vi "Temperature Limit.vi"(3 "Limite supérieure":dbl=80.0 format="%.2f", 4 "delta t (ms)":u32=400 min=50 max=2000 step=50, 5 "Points à acquérir":i32=75 min=20 max=500) -> ()   [LabVIEW 2013]
doc: "Ce VI simule l'acquisition de température, trace la température et notifie l'utilisateur si la température dépasse la limite."
panel:
  out "Limite dépassée":bool
  in  "Abandonner":bool
  out "Température":cluster{"Temperature":dbl, "High Limit":dbl}(graph)
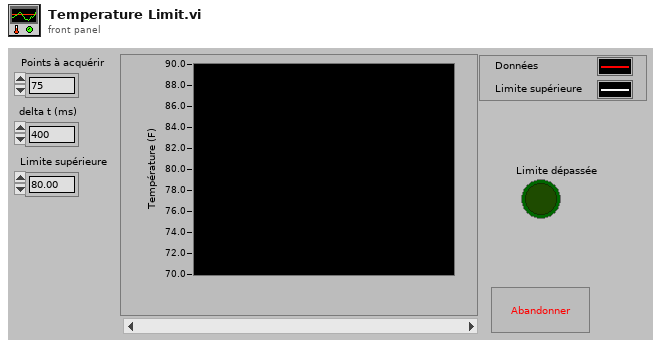
[diagram p1: front panel]
types:
  T1 = cluster{"Température":dbl, "Limite supérieure":dbl}
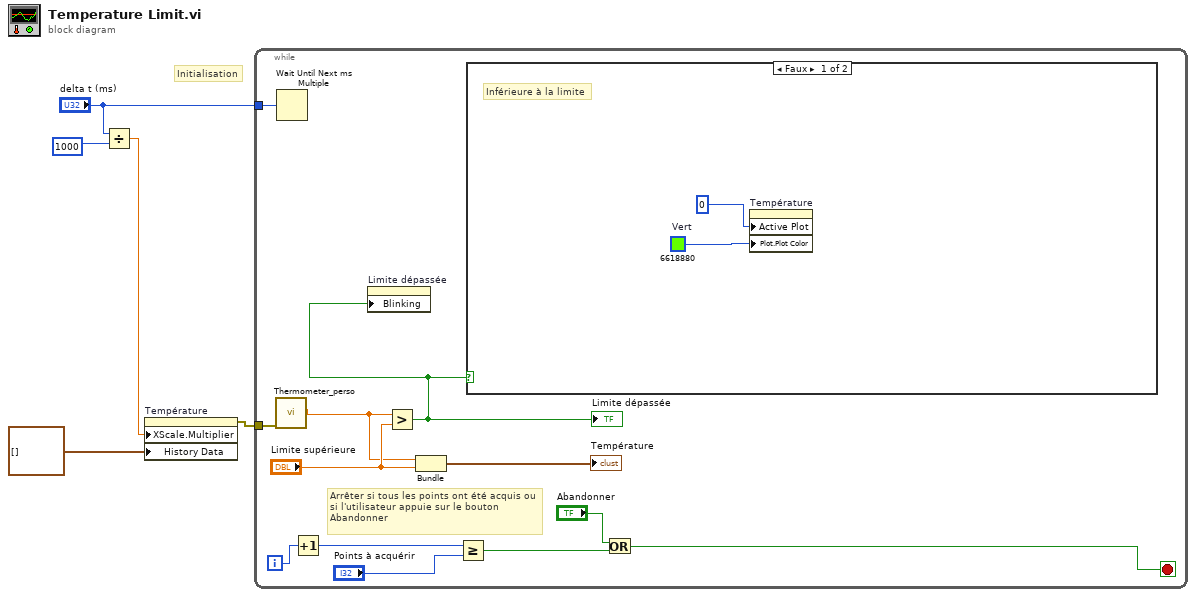
[diagram p0: block diagram]
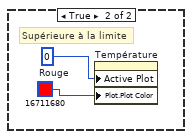
[diagram p2: hidden frame]
diagram:
  # "Initialisation"
  n1 = Divide(x="delta t (ms)", y=1000) -> (x/y=w3:dbl)
  n2 = property on="Température" class="GraphDér (strict)"("XScale.Multiplier"=w3, "History Data"=cluster{"Temperature":dbl, "High Limit":dbl}[] [] ("Données d'historique")) -> (error out=w2:errorcluster)  [unwired: 2 in, 1 out]
  n3 = while "Boucle While" {
    tunnel: "delta t (ms)" -> [w9]
    tunnel: w2 -> [w7]
    i -> [w16]
    stop <- w10 stop-if-true
    # "Supérieure à la limite"
    # "Arrêter si tous les points ont été acquis ou si l'utilisateur appuie sur le bouton Abandonner"
    n4 = call "Thermometer_perso.vi"("entrée d'erreur (pas d'erreur)"=w7) -> ("Température"=w8:dbl)  [unwired: 9 in, 1 out]
    n5 = Wait Until Next ms Multiple ("Structure Séquence empilée")(millisecond multiple=w9) -> ()  [unwired: 1 out]
    n6 = Increment ("Incrémenter")(x=w16) -> (x+1=w14:i32)
    n7 = Greater? ("Déplacer")(x=w8, y="Limite supérieure") -> (0:w6:bool)
    "Limite dépassée" <- w6
    n8 = property on="Limite dépassée" class="Bool (strict)"("Blinking"=w6) -> ()  [unwired: 2 in, 2 out]
    n9 = Bundle ("Rotation")("Température"=w8, "Limite supérieure"="Limite supérieure") -> (→"Température":T1)  [unwired: 1 in]
    n10 = Greater Or Equal? ("Supérieur ou égal ?")(x=w14, y="Points à acquérir") -> (x >= y?=w12:bool)
    n11 = case "Structure Condition" shown="Faux" w6 {
      frame False {
        w18 = u32 6618880  # Vert
        # "Inférieure à la limite"
        n12 = property on="Température" class="GraphDér (strict)"("Active Plot"=0, "Plot.Plot Color"=w18) -> ()  [unwired: 2 in, 2 out]
      }
      frame True {
        w21 = u32 16711680  # Rouge
        # "Supérieure à la limite"
        n13 = property on="Température" class="GraphDér (strict)"("Active Plot"=0, "Plot.Plot Color"=w21) -> ()  [unwired: 2 in, 2 out]
      }
    }
    n14 = Or ("OU")(x="Abandonner", y=w12) -> (x .or. y?=w10:bool)
  }
